vi "Init CCD monitor Config Obj by Label.vi"(8 "error in (no error)":errorcluster, 10 "Label":string, 11 "Hardware.lvlib:CCD monitor.lvlib:CCD monitor configuration.lvclass":refnum<class "CCD monitor configuration.lvclass">) -> (0 "error out":errorcluster, 1 "not found?":bool, 2 "Hardware.lvlib:CCD.lvlib:CCD Configuration.lvclass":refnum<class "CCD Configuration.lvclass">, 3 "reference out":refnum<class "CCD monitor configuration.lvclass">)   [LabVIEW 2016, in "CCD monitor.lvlib" / "CCD monitor configuration.lvclass"]
uses:
  <userlib>/Common Components/Hardware/Abstract System/Monitor/CCD monitor configuration.lvclass
  <userlib>/Common Components/Hardware/Abstract System/Monitor/CCD monitor.lvclass
  <userlib>/Common Components/Hardware/CCD/CCD Configuration.lvclass
  <userlib>/Common Components/Hardware/CCD/CCD/CCD.lvclass
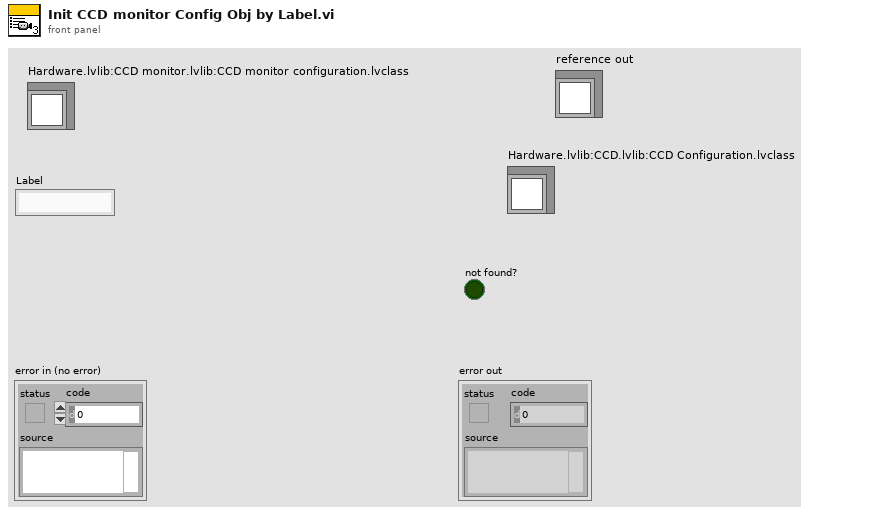
[diagram p1: front panel]
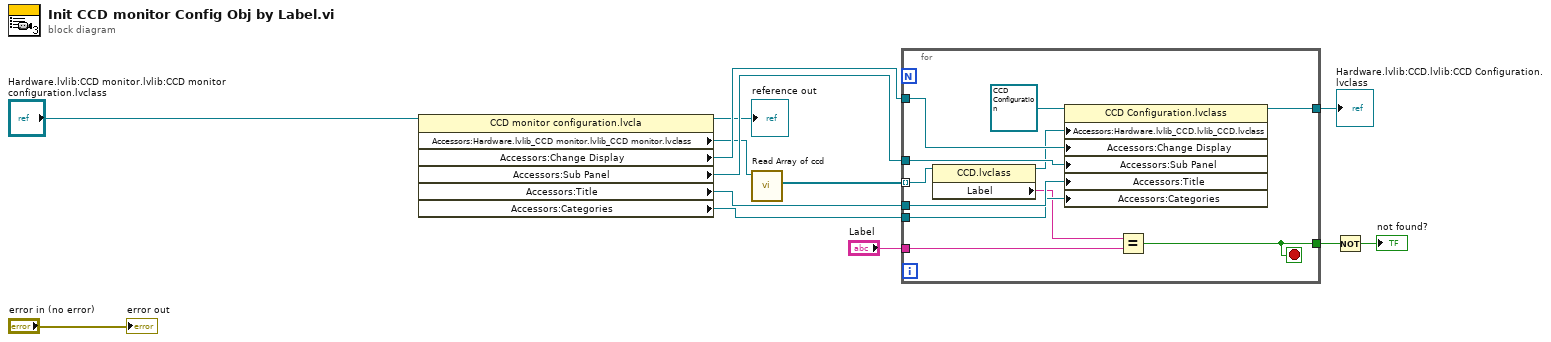
[diagram p0: block diagram]
diagram:
  n1 = property class="CCD monitor configuration.lvcla"(reference="Hardware.lvlib:CCD monitor.lvlib:CCD monitor configuration.lvclass") -> (reference out=→"reference out":refnum<class "CCD monitor configuration.lvclass">, "Accessors:Hardware.lvlib_CCD monitor.lvlib_CCD monitor.lvclass"=w3:refnum<class "CCD monitor.lvclass">, "Accessors:Change Display"=w12:refnum<user-event>, "Accessors:Sub Panel"=w11:refnum<vi>, "Accessors:Title"=w10:refnum<vi>, "Accessors:Categories"=w9:refnum<vi>)  [unwired: 1 in, 1 out]
  n2 = call <userlib>:"Read Array of ccd.vi"("CCD monitor in"=w3) -> ("Array of ccd"=w2:refnum<class "CCD.lvclass">[])  [unwired: 9 in, 1 out]
  n3 = for {
    tunnel: w12 -> [w24]
    tunnel: w11 -> [w23]
    tunnel: w10 -> [w22]
    tunnel: w9 -> [w21]
    tunnel: "Label" -> [w18]
    tunnel: [w17] -> w1
    tunnel: [w16] -> w7
    tunnel: w2 -> [w14] mode=indexing
    stop <- w16 stop-if-true
    n4 = property class="CCD.lvclass"(reference=w14) -> (reference out=w20:refnum<class "CCD.lvclass">, "Label"=w19:string)  [unwired: 1 in, 1 out]
    n5 = property class="CCD Configuration.lvclass"(reference=refnum<class "CCD Configuration.lvclass"> refnum ("Hardware.lvlib:CCD.lvlib:CCD Configuration.lvclass"), "Accessors:Hardware.lvlib_CCD.lvlib_CCD.lvclass"=w20, "Accessors:Change Display"=w24, "Accessors:Sub Panel"=w23, "Accessors:Title"=w22, "Accessors:Categories"=w21) -> (reference out=w17:refnum<class "CCD Configuration.lvclass">)  [unwired: 1 in, 1 out]
    n6 = Equal?(x=w19, y=w18) -> (x = y?=w16:bool)
  }
  "Hardware.lvlib:CCD.lvlib:CCD Configuration.lvclass" <- w1
  n7 = Not(x=w7) -> (.not. x?=→"not found?":bool)
  "error out" <- "error in (no error)"
